vi "qRTR.vi"(0 "System no.":i32=1 min=1 max=4 step=1, 5 "error in":errorcluster) -> (14 "Record table rate":i32, 19 "error out":errorcluster)   [LabVIEW 2020]
doc: "Returns the current table rate.\n\nC-887, F-206, M-8X0: Only for GCS syntax version = GCS 2.0 or higher (check with CSV?.vi. If CSV?.vi is not supported, syntax version is GCS 1.0)."
panel:
  # "Returns the current table rate."
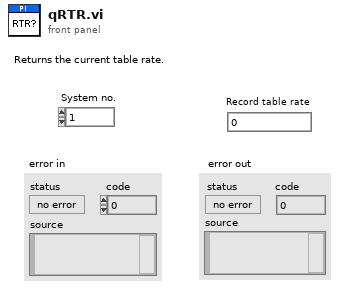
[diagram p1: front panel]
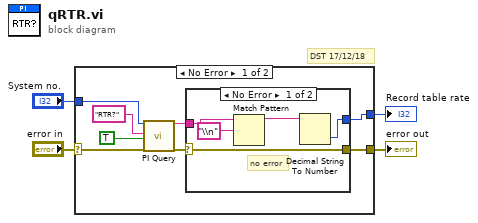
[diagram p0: block diagram]
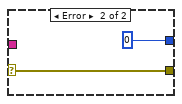
[diagram p2: hidden frame]
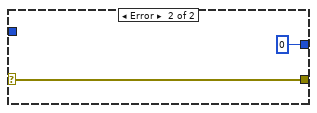
[diagram p3: hidden frame]
diagram:
  # "DST 17/12/18"
  n1 = case shown="No Error" "error in" {
    selector: "error in" -> [w5 w21]
    tunnel: [w12 0] -> w4
    tunnel: "System no." -> [w10 _]
    tunnel: [w7 w21] -> w2
    frame No Error {
      n2 = call "PI Query.vi"("System no."=w10, "String to send"="RTR?", "Attach termination char.?"=TRUE ("Attach Linefeed?"), "error in"=w5) -> ("String read"=w8:string, "error out"=w6:errorcluster)  [unwired: 3 in, 11 out]
      n3 = case shown="No Error" w6 {
        selector: w6 -> [w13 w18]
        tunnel: w8 -> [w16 _]
        tunnel: [w17 0] -> w12
        tunnel: [w13 w18] -> w7
        frame No Error {
          # "no error"
          n4 = Match Pattern(string=w16, regular expression="\\n") -> (before substring=w14:string)  [unwired: 4 out]
          n5 = Decimal String To Number(string=w14) -> (number=w17:i32)  [unwired: 3 out]
        }
        frame Error {
        }
      }
    }
    frame Error {
    }
  }
  "error out" <- w2
  "Record table rate" <- w4
